vi "LSA.vi"() -> ()   [LabVIEW 2018]
uses:
  wlmData.dll
panel:
  out "error out":errorcluster
  in  "Channel":i32
  out "wavelength / nm":dbl format="%#_18f"
  in  "stop":bool
  out "wavelength graph":dbl[](graph)
  out "power graph":dbl[](graph)
  out "Power":dbl
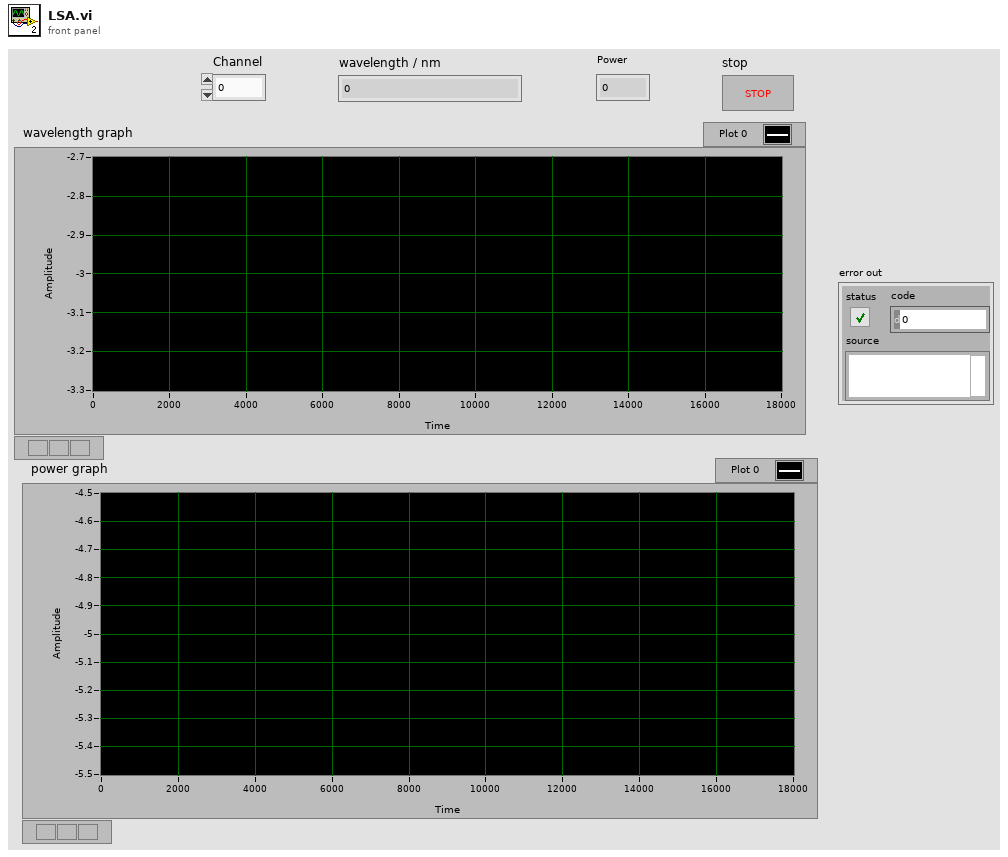
[diagram p1: front panel]
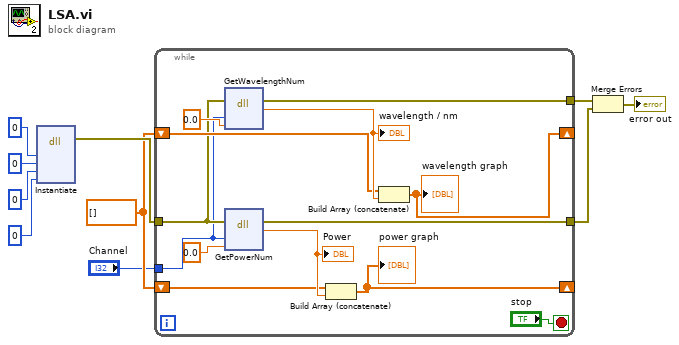
[diagram p0: block diagram]
diagram:
  w6 = dbl[] []
  n1 = dll-call lib="wlmData.dll" fn="Instantiate"("arg1"=u32 0, "arg2"=0, "arg3"=u32 0, "arg4"=u32 0) -> (error out=w7:errorcluster)  [unwired: 8 in, 1 out]
  n2 = while {
    tunnel: w7 -> [w18]
    shift-right: [w19] -> _
    shift-left: w6 -> [w20]
    shift-right: [w14] -> _
    shift-left: w6 -> [w15]
    tunnel: "Channel" -> [w13]
    tunnel: [w12] -> w3
    tunnel: [w11] -> w2
    stop <- "stop" stop-if-true
    n3 = dll-call lib="wlmData.dll" fn="GetWavelengthNum"(error in=w18, "arg1"=w13, "arg2"=0.0) -> (error out=w12:errorcluster, "return type"=w21:dbl)  [unwired: 4 in, 1 out]
    "wavelength / nm" <- w21
    n4 = dll-call lib="wlmData.dll" fn="GetPowerNum"(error in=w18, "arg1"=w13, "arg2"=0.0) -> (error out=w11:errorcluster, "return type"=w16:dbl)  [unwired: 4 in, 1 out]
    "Power" <- w16
    n5 = Build Array (concatenate)(w15, w16) -> (w14:dbl[])
    "power graph" <- w14
    n6 = Build Array (concatenate)(w20, w21) -> (w19:dbl[])
    "wavelength graph" <- w19
  }
  n7 = Merge Errors(w3, w2) -> (→"error out":errorcluster)
